vi "test14-Interrupt_Event.vi"(8 "error in (no error)":errorcluster, 11 "TestCase in":refnum<class "testcase-CSMGlobalLog.lvclass">) -> (0 "error out":errorcluster, 3 "TestCase out":refnum<class "testcase-CSMGlobalLog.lvclass">)   [LabVIEW 2017, in "testcase-CSMGlobalLog.lvclass"]
uses:
  testcase-CSMGlobalLog.lvclass
  testcase-CSMGlobalLog.lvclass/testcase-CSMGlobalLog.ctl
  src/user.lib/_NEVSTOP/Communicable State Machine(CSM)/_Support/Typedef/_CSM_GlobalLog_MSG.ctl
  src/user.lib/_NEVSTOP/Communicable State Machine(CSM)/_Support/Typedef/_CSM_Response Source Message.ctl
  src/user.lib/_NEVSTOP/Communicable State Machine(CSM)/_Support/Typedef/_CSM_GlobalLog_MSG_TYPE.ctl
  26934866-e646-479d-ab77-64683b41bd31.vi
  d7fa9ef8-312d-468d-b02b-a1c2fcb7fbb3.vi
  c0dc643a-0362-49fc-99f4-5251266ba5a0.vi
  src/user.lib/_NEVSTOP/Communicable State Machine(CSM)/_Support/GlobalEvent/GEvt-Generate with Rule Check.vi
  src/user.lib/_NEVSTOP/Communicable State Machine(CSM)/AdvanceAPI/CSM - Convert Error to Argument.vi
  src/user.lib/_NEVSTOP/Communicable State Machine(CSM)/_Support/GlobalEvent/Cache-GEvt Refs.vi
  src/user.lib/_NEVSTOP/Communicable State Machine(CSM)/AdvanceAPI/CSM - Make String Arguments Safe.vi
  src/user.lib/_NEVSTOP/Communicable State Machine(CSM)/_Support/ChangeFlag/FlagInstance-GEvt Refs.vi
  src/user.lib/_NEVSTOP/Communicable State Machine(CSM)/AdvanceAPI/CSM - Keywords.vi
  src/user.lib/_NEVSTOP/Communicable State Machine(CSM)/_Support/ChangeFlag/ChangeFlag-Read.vi
  src/user.lib/_NEVSTOP/Communicable State Machine(CSM)/_Support/ChangeFlag/ChangeFlagDB.vi
  src/user.lib/_NEVSTOP/Communicable State Machine(CSM)/_Support/GlobalEvent/FGV-GlobalEventRef(lvlibp).vi
  src/user.lib/_NEVSTOP/Communicable State Machine(CSM)/_Support/GlobalEvent/FGV-GlobalEventQueues(lvlibp).vi
  src/user.lib/_NEVSTOP/Communicable State Machine(CSM)/_Support/GlobalEvent/GEvt-Valid Subscribers.vi
  src/user.lib/_NEVSTOP/Communicable State Machine(CSM)/_Support/GlobalEvent/LogFilter/LogFilter - Check.vi
  src/user.lib/_NEVSTOP/Communicable State Machine(CSM)/_Support/GlobalEvent/LogFilter/LogFilter.lvclass
  <vilib>/addons/_JKI Toolkits/VI Tester/TestCase.llb/TestCase.lvclass
  src/user.lib/_NEVSTOP/Communicable State Machine(CSM)/Communicable State Machine.lvlib
  C:/Program Files (x86)/National Instruments/LabVIEW 2017/vi.lib/addons/_JKI Toolkits/VI Tester/TestCase.llb/TestCase.lvclass
panel:
  out "String cache each loop":string
  out "LoopCount":i32
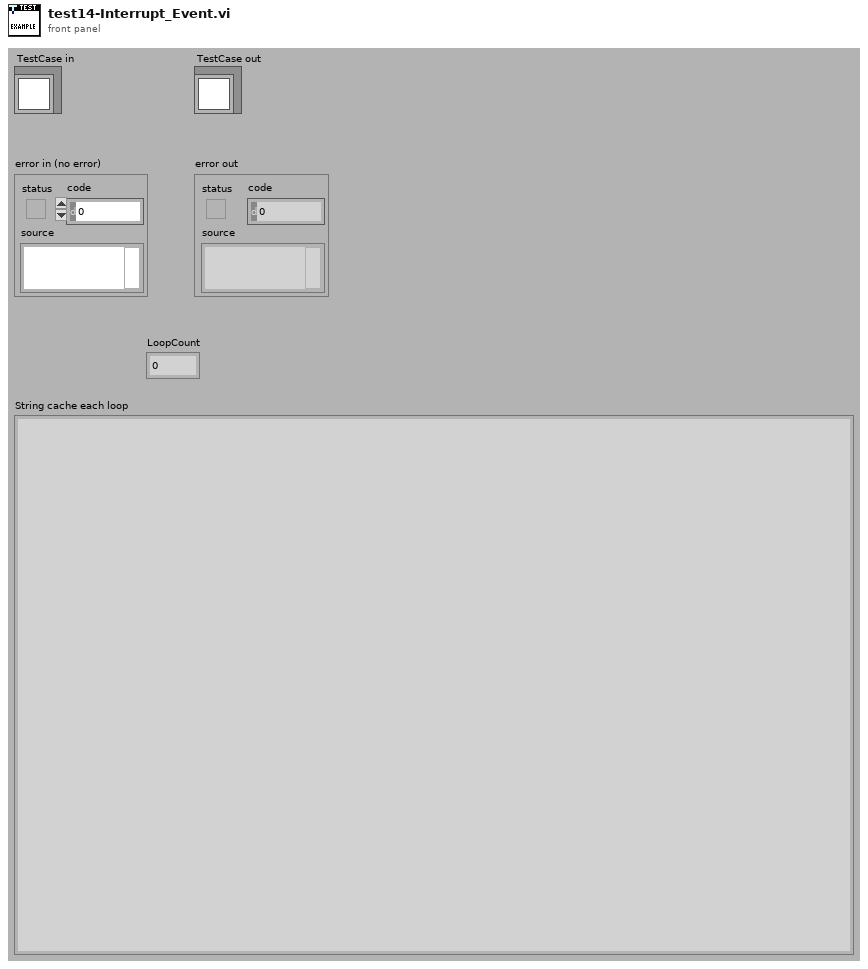
[diagram p1: front panel]
types:
  T1 = typedef "Communicable State Machine.lvlib/_CSM_GlobalLog_MSG.ctl" = cluster{"Name (\"\" to Use UUID)":string, "Current State":string, "Arguments":string, "Source Message":T2, "Source Module":string, "Complete(T)/Start(F)":bool, "LogType":T3, "Time Stamp":timestamp}
  T2 = typedef "Communicable State Machine.lvlib/_CSM_Response Source Message.ctl" = cluster{"‘State":string, "’Arguments":string, "’Error":errorcluster}
  T3 = typedef "Communicable State Machine.lvlib/_CSM_GlobalLog_MSG_TYPE.ctl" = enum16{"User Log", "State Change", "Status", "Interrupt", "Register", "Unregister", "Error Log", "Module Created", "Module Destroyed", "Async Message", "No-Rep Async Message", "Sync Message"}
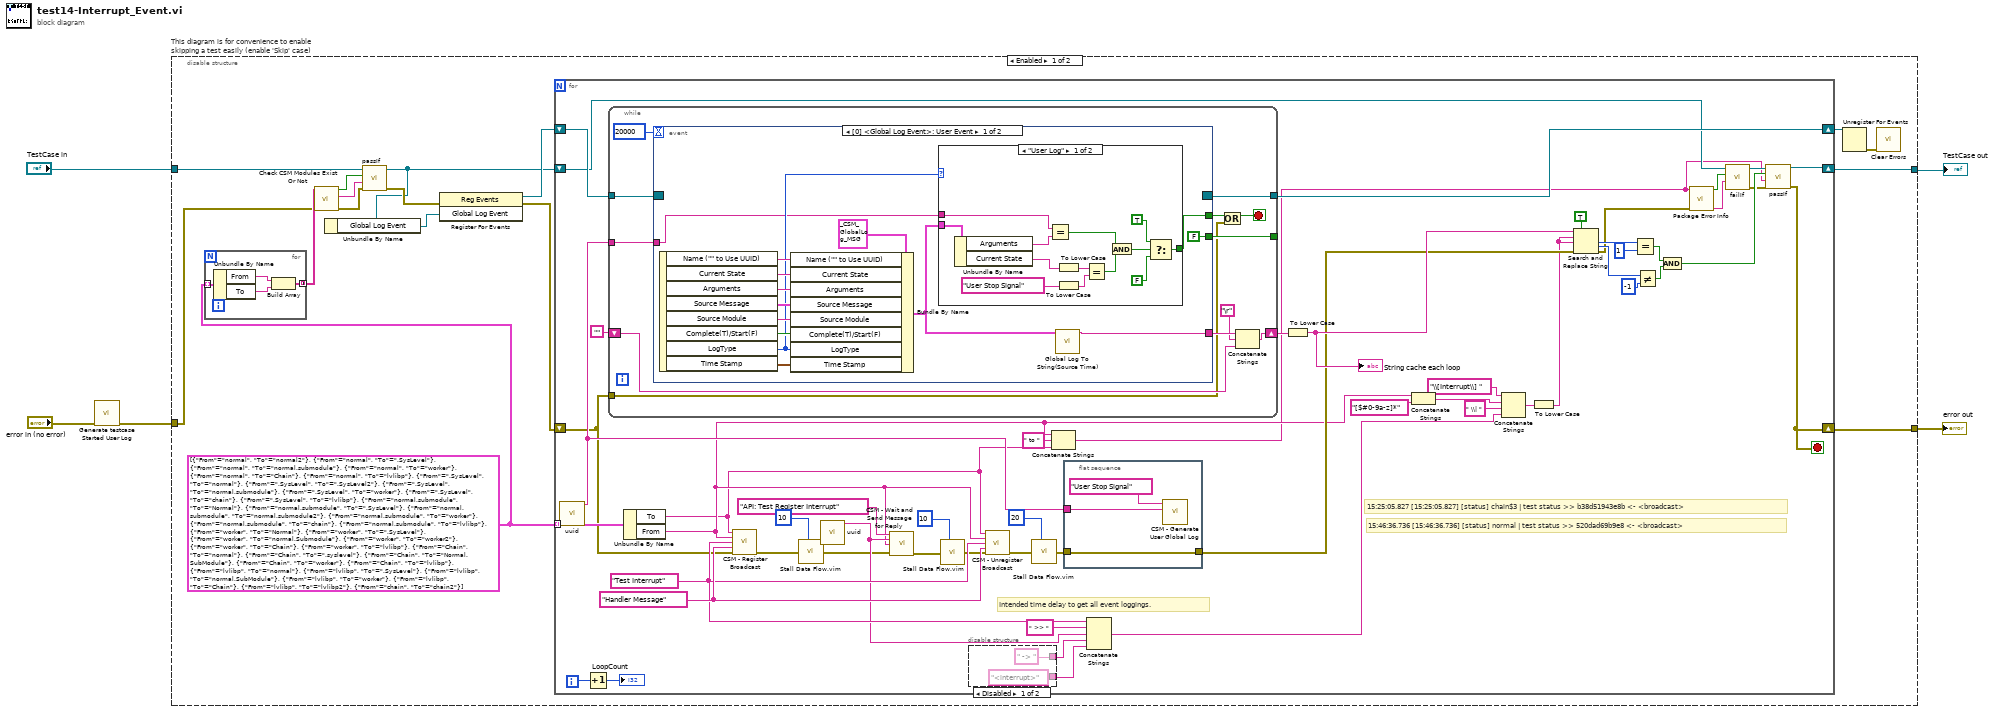
[diagram p0: block diagram]
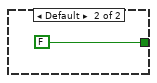
[diagram p3: hidden frame]
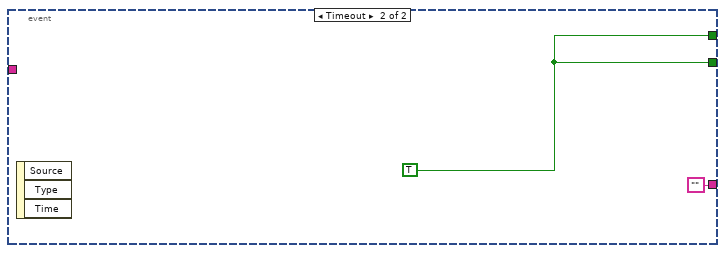
[diagram p4: hidden frame]
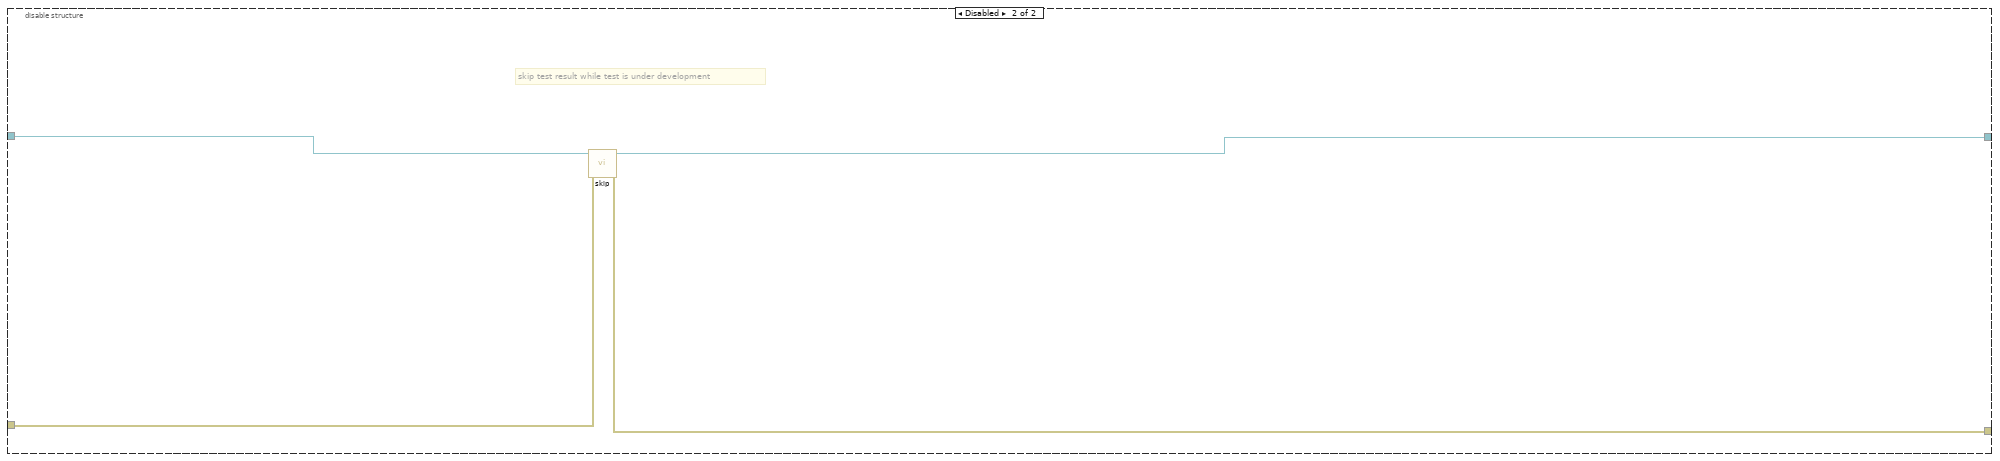
[diagram p5: hidden frame]
diagram:
  n1 = call "Generate testcase Started User Log.vi"("Error In"="error in (no error)") -> ("error out"=w1:errorcluster)  [unwired: 10 in]
  n2 = disable-structure "This diagram is for convenience to enable skipping a test easily (enable 'Skip' case)" shown="Enabled" {
    disable-tunnel: "TestCase in" -> [w12 w130]
    disable-tunnel: [w18 w128] -> w2
    disable-tunnel: [w17 w129] -> w4
    disable-tunnel: w1 -> [w10 w127]
    frame Enabled {
      w9 = cluster{"From":string, "To":string}[] [{"From"="normal", "To"="normal2"}, {"From"="normal", "To"=".SysLevel"}, {"From"="normal", "To"="normal.submodule"}, {"From"="normal", "To"="worker"}, {"From"="normal", "To"="Chain"}, {"From"="normal", "To"="lvlibp"}, {"From"=".SysLevel", "To"="normal"}, {"From"=".SysLevel", "To"=".SysLevel2"}, {"From"=".SysLevel", "To"="normal.submodule"}, {"From"=".SysLevel", "To"="worker"}, {"From"=".SysLevel", "To"="chain"}, {"From"=".SysLevel", "To"="lvlibp"}, {"From"="normal.submodule", "To"="Normal"}, {"From"="normal.submodule", "To"=".SysLevel"}, {"From"="normal.submodule", "To"="normal.submodule2"}, {"From"="normal.submodule", "To"="worker"}, {"From"="normal.submodule", "To"="chain"}, {"From"="normal.submodule", "To"="lvlibp"}, {"From"="worker", "To"="Normal"}, {"From"="worker", "To"=".SysLevel"}, {"From"="worker", "To"="normal.Submodule"}, {"From"="worker", "To"="worker2"}, {"From"="worker", "To"="Chain"}, {"From"="worker", "To"="lvlibp"}, {"From"="Chain", "To"="normal"}, {"From"="Chain", "To"=".syslevel"}, {"From"="Chain", "To"="Normal.SubModule"}, {"From"="Chain", "To"="worker"}, {"From"="Chain", "To"="lvlibp"}, {"From"="lvlibp", "To"="normal"}, {"From"="lvlibp", "To"=".SysLevel"}, {"From"="lvlibp", "To"="normal.SubModule"}, {"From"="lvlibp", "To"="worker"}, {"From"="lvlibp", "To"="Chain"}, {"From"="lvlibp", "To"="lvlibp2"}, {"From"="chain", "To"="chain2"}]
      n3 = for {
        tunnel: w9 -> [w25] mode=indexing
        tunnel: [w22] -> w15 mode=concatenating
        n4 = Unbundle By Name(w25) -> ("From"=w24:string, "To"=w23:string)
        n5 = Build Array(w24, w23) -> (w22:string[])
      }
      n6 = call "Check CSM Modules Exist Or Not.vi"("error in"=w10, "CSM names in"=w15) -> ("error out"=w13:errorcluster, "Debug string"=w14:string, "All Modules Exist?"=w16:bool)  [unwired: 7 in]
      n7 = call-dynamic "passIf.vi"("error in (no error)"=w13, "message (\"\")"=w14, "pass"=w16, "TestCase in"=w12) -> ("error out"=w11:errorcluster, "TestCase out"=w8:refnum<class "testcase-CSMGlobalLog.lvclass">)  [unwired: 6 in]
      n8 = Unbundle By Name(w8) -> ("Global Log Event"=w7:refnum<user-event>)
      n9 = register-events(error in=w11, w7) -> (reference out=w21:refnum<event-registration>, error out=w19:errorcluster)  [unwired: 1 in]
      n10 = for {
        shift-right: [w78] -> w20
        shift-left: w21 -> [w79]
        shift-right: [w75] -> w17
        shift-left: w19 -> [w42]
        tunnel: w9 -> [w56] mode=indexing
        shift-right: [w77] -> w18
        shift-left: w8 -> [w40]
        i -> [w64]
        stop <- w75 stop-if-true
        w59 = "Handler Message" ("API (If \"\", Same as Trigger)")
        w52 = "Test Interrupt" ("Trigger")
        # "15:46:36.736 [15:46:36.736] [status] normal | test status >> 520dad69b9e8 <- <broadcast>"
        # "15:25:05.827 [15:25:05.827] [status] chain$3 | test status >> b38d51943e8b <- <broadcast>"
        # "Intended time delay to get all event loggings."
        n11 = call "uuid.vi"() -> ("UUID"=w65:string)  [unwired: 11 in]
        n12 = Increment(x=w64) -> (x+1=→"LoopCount":i32)
        n13 = while {
          tunnel: w79 -> [w96]
          tunnel: [w95] -> w78
          shift-right: [w87] -> w60
          shift-left: "" -> [w90]
          tunnel: w65 -> [w92]
          tunnel: [w91] -> _
          tunnel: w42 -> [w85]
          stop <- w86 stop-if-true
          n14 = event shown="[0] <Global Log Event>: User Event" {
            selector: w96 -> [_ _]
            dyn-events: [_ _] -> w95
            timeout: 20000 -> [_ _]
            tunnel: [w97 ""] -> w89
            tunnel: [w99 w126] -> w94
            tunnel: w92 -> [w100 _]
            tunnel: [FALSE ("Stop") w126] -> w91
            event User Event {
              n15 = event-data() -> ("Name (\"\" to Use UUID)"=w109:string, "Current State"=w108:string, "Arguments"=w107:string, "Source Message"=w106:T2, "Source Module"=w105:string, "Complete(T)/Start(F)"=w104:bool, "LogType"=w101:T3, "Time Stamp"=w103:timestamp)  [unwired: 1 in]
              n16 = Bundle By Name(cluster=T1 {"Name (\"\" to Use UUID)"="", "Current State"="", "Arguments"="", "Source Message"={"‘State"="", "’Arguments"="", "’Error"={"status"=FALSE, "code"=0, "source"=""}}, "Source Module"="", "Complete(T)/Start(F)"=FALSE, "LogType"=enum."State Change", "Time Stamp"=timestamp(0 s since 1904-01-01)} ("Cross CSM Data"), "Name (\"\" to Use UUID)"=w109, "Current State"=w108, "Arguments"=w107, "Source Message"=w106, "Source Module"=w105, "Complete(T)/Start(F)"=w104, "LogType"=w101, "Time Stamp"=w103) -> (w98:T1)
              n17 = case shown="\"User Log\"" w101 {
                tunnel: w98 -> [w123 _]
                tunnel: w100 -> [w122 _]
                tunnel: [w111 FALSE] -> w99
                frame "User Log" {
                  n18 = Unbundle By Name(w123) -> ("Arguments"=w121:string, "Current State"=w120:string)
                  n19 = Equal?(x=w122, y=w121) -> (x = y?=w115:bool)
                  n20 = To Lower Case(string=w120) -> (all lower case string=w119:string)
                  n21 = To Lower Case(string="User Stop Signal" ("Log")) -> (all lower case string=w117:string)
                  n22 = Equal?(x=w119, y=w117) -> (x = y?=w116:bool)
                  n23 = And(x=w115, y=w116) -> (x .and. y?=w114:bool)
                  n24 = Select(t=TRUE, s=w114, f=FALSE) -> (s? t:f=w111:bool)
                }
                frame Default {
                }
              }
              n25 = call "Global Log To String(Source Time).vi"("Log"=w98) -> ("Log String"=w97:string)  [unwired: 9 in]
            }
            event Timeout {
              w126 = TRUE ("Stop")
              n26 = event-data() -> ()  [unwired: 1 in, 3 out]
            }
          }
          n27 = Or(x=w94, y=w85) -> (x .or. y?=w86:bool)
          n28 = Concatenate Strings(w89, "\r", w90) -> (w87:string)
        }
        n29 = Unbundle By Name(w56) -> ("To"=w34:string, "From"=w35:string)
        n30 = call "CSM - Register Broadcast.vi"("CSM Name(Empty for Broadcast Event)"=w34, "Source CSM Name (* as Default)"=w35, "Trigger"=w52, "API (If \"\", Same as Trigger)"=w59, "Error In"=w42) -> ("error out"=w27:errorcluster)  [unwired: 9 in, 1 out]
        n31 = call "Stall Data Flow.vim"("value in"=w27, "milliseconds to wait"=u32 10) -> ("value out"=w26:errorcluster)  [unwired: 1 out]
        n32 = call "uuid.vi"() -> ("UUID"=w51:string)  [unwired: 11 in]
        n33 = call "CSM - Wait and Send Message for Reply.vi"("State"="API: Test Register Interrupt", "Arguments (\"\")"=w51, "Target Module"=w35, "Error In (No Error)"=w26) -> ("error out"=w31:errorcluster)  [unwired: 8 in, 3 out]
        n34 = call "Stall Data Flow.vim"("value in"=w31, "milliseconds to wait"=u32 10) -> ("value out"=w30:errorcluster)  [unwired: 1 out]
        n35 = disable-structure shown="Disabled" {
          disable-tunnel: [" -> " ("string") _] -> w54
          disable-tunnel: ["<interrupt>" ("search string") _] -> w53
          frame Disabled {
          }
          frame Enabled {
          }
        }
        n36 = call "CSM - Unregister Broadcast.vi"("CSM Name(Empty for Broadcast Event)"=w34, "Source CSM Name (* as Default)"=w35, "Trigger"=w52, "API (\"*\" as Default)"=w59, "Error In"=w30) -> ("error out"=w57:errorcluster)  [unwired: 9 in, 1 out]
        n37 = call "Stall Data Flow.vim"("value in"=w57, "milliseconds to wait"=u32 20) -> ("value out"=w66:errorcluster)  [unwired: 1 out]
        n38 = Concatenate Strings(w35, " to " ("string"), w34) -> (w32:string)
        n39 = flat-sequence {
          tunnel: w65 -> [w83]
          tunnel: w66 -> [w82]
          tunnel: [w82] -> w61
          frame #0 {
            n40 = call "CSM - Generate User Global Log.vi"("Arguments"=w83, "Log"="User Stop Signal") -> ()  [unwired: 9 in, 1 out]
          }
        }
        n41 = Concatenate Strings(w52, " >> " ("string"), w51, w54, w53) -> (w44:string)
        n42 = To Lower Case(string=w60) -> (all lower case string=w62:string)
        "String cache each loop" <- w62
        n43 = Concatenate Strings(w35, "[$#0-9a-z]*" ("string")) -> (w45:string)
        n44 = Concatenate Strings("\\[Interrupt\\] " ("regular expression"), w45, " \\| " ("string"), w44) -> (w48:string)
        n45 = To Lower Case(string=w48) -> (all lower case string=w43:string)
        n46 = Search and Replace String(replace all?=TRUE ("replace all? (F)"), input string=w62, search string=w43, replace string=w43, error in=w61) -> (number of replacements=w71:i32, offset past replacement=w72:i32, error out=w36:errorcluster)  [unwired: 3 in, 1 out]
        n47 = Equal?(x=w71, y=1) -> (x = y?=w73:bool)
        n48 = Not Equal?(x=w72, y=-1) -> (x != y?=w74:bool)
        n49 = And(x=w73, y=w74) -> (x .and. y?=w50:bool)
        n50 = call "Package Error Info.vi"("error in"=w36, "String in"=w32) -> ("packed error info out"=w39:string, "error status"=w41:bool)  [unwired: 8 in]
        n51 = call-dynamic "failIf.vi"("message (\"\")"=w39, "fail"=w41, "TestCase in"=w40) -> ("error out"=w37:errorcluster, "TestCase out"=w38:refnum<class "testcase-CSMGlobalLog.lvclass">)  [unwired: 7 in]
        n52 = call-dynamic "passIf.vi"("error in (no error)"=w37, "message (\"\")"=w32, "pass"=w50, "TestCase in"=w38) -> ("error out"=w75:errorcluster, "TestCase out"=w77:refnum<class "testcase-CSMGlobalLog.lvclass">)  [unwired: 6 in]
      }
      n53 = Unregister For Events(event registration refnum=w20) -> (error out=w6:errorcluster)  [unwired: 1 in]
      n54 = call <vilib>:"Clear Errors.vi"("error in (no error)"=w6) -> ()  [unwired: 5 in, 2 out]
    }
    frame Disabled {
      # "skip test result while test is under development"
      n55 = call <vilib>:"skip.vi"("error in (no error)"=w127, "TestCase in"=w130) -> ("error out"=w129:errorcluster, "TestCase out"=w128:refnum<class "testcase-CSMGlobalLog.lvclass">)  [unwired: 8 in]
    }
  }
  "error out" <- w4
  "TestCase out" <- w2
